vi "Test Initiate.vi"(0 "Template Tx Test in":refnum<class "niDTS BT Tx Test.lvclass">, 11 "error in (no error)":errorcluster) -> (4 "Template Tx Test out":refnum<class "niDTS BT Tx Test.lvclass">, 15 "error out":errorcluster)   [LabVIEW 2015, in "niDTS BT.lvlib" / "niDTS BT Tx Test.lvclass"]
uses:
  niDTS BT Tx Test.lvclass
  niDTS BT Tx Test.lvclass/niDTS BT Tx Test.ctl
  Instrument/INSTR TX/niDTS BT INSTR TX.lvclass
  Framework/Dut/Objects/BASE_class/niDTS Dut.lvclass
  RiviInstDriver/niRfsaBT/Objects/niRfsaBt.lvclass
  niDTS BT.lvlib
  Dut/Objects/BASE_class/niDTS BT Dut.lvclass
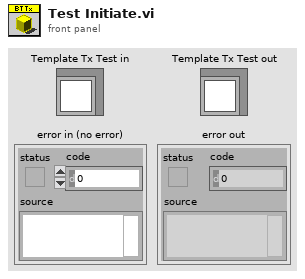
[diagram p1: front panel]
types:
  T1 = typedef "niDTS BT.lvlib/niDTS BT Tx Test INC Parameters.ctl" = cluster{"Channel":i32, "Data Rate ":i32, "Dut Tx Power":dbl, "External Attenuation (dB)":dbl[], "Auto Level":bool, "Packet type":T2, "Payload Pattern":T3, "Burst Sync":enum16{"NONE", "PREamble"}, "BD ADDRESS":u32, "Packet Length, bytes":i32, "ModAcc Measurement Paramaters":cluster{"ModAcc Enable":bool, "CFO Enable":bool, "Character Select":T4, "Averages":i32, "Averaging Mode":enum16{"RMS", "LOG", "SCALAR", "MAX", "MIN", "VECTOR"}, "Measurement Length":i32, "Measurement Offset":i32}, "OBW Measurement Parameters":T5, "TXP Measurement Parameters":T6, "IBE  Measurement Parameters":T7, "Trace Enable":bool, "Trigger":T8}
  T2 = typedef "niDTS BT.lvlib/niDTS BT INC Packet Type.ctl" = enum16{"NULL", "POLL", "FHS", "DM1", "DH1", "HV1", "HV2", "HV3", "EV3", "DV", "AUX1", "DM3", "DH3", "EV4", "EV5", "DM5", "DH5", "LE-TP"}
  T3 = typedef "niDTS BT.lvlib/niDTS BT Tx Test INC BD Payload Data.ctl" = enum16{"0", "1", "01", "00001111", "PN9", "AUTO"}
  T4 = typedef "niDTS BT.lvlib/niDTS BT Tx Test INC Modulation Characteristics.ctl" = enum16{"DF1", "DF2", "BOTH"}
  T5 = typedef "niDTS BT.lvlib/niDTS BT INC OBW Measurement Parameters.ctl" = cluster{"OBW Enable":bool, "OBW Averages":i32, "Averaging Type":enum16{"RMS", "LOG", "SCALAR", "MAX", "MIN", "VECTOR"}, "Measurement Interval Mode":enum16{"AUTO", "MANUAL"}, "Measurement Interval Length (sec)":dbl}
  T6 = typedef "niDTS BT.lvlib/niDTS BT INC TXP Measurement Parameters.ctl" = cluster{"TXP Power Enable":bool, "TXP Averages":i32, "Averaging Type":enum16{"RMS", "LOG", "SCALAR", "MAX", "MIN"}}
  T7 = typedef "niDTS BT.lvlib/niDTS BT INC EDR IBE Measurement Parameters.ctl" = cluster{"IBE Enable":bool, "IBE Averages":i32, "Averaging Type":enum16{"RMS", "LOG", "SCALAR", "MAX", "MIN", "VECTOR"}, "Numbe of Channels":i32, "Channel Mode":enum16{"InBand", "Centered"}, "Measurement Interval Mode":enum16{"AUTO", "MANUAL"}, "Measurement Interval Length (sec)":dbl}
  T8 = typedef "niDTS BT.lvlib/niDTS BT DUT INC Trigger.ctl" = cluster{"MinQuietTimeDuration (sec)":dbl, "TriggerDelay (sec)":dbl, "TriggerEdge":enum16{"RISing", "FALLing"}, "TriggerSource":enum16{"IMMediate", "RF0", "PFI0", "PFI1", "RTS0", "RTS1", "RTS2", "RTS3", "RTS4", "RTS5", "RTS6", "RTS7", "PXIStar", "SOFT"}, "TriggerThreshold (dB)":dbl, "TriggerTimeout (sec)":dbl}
  T9 = typedef "niDTS Framework.lvlib/niDTS Dut INC Handle.ctl" = refnum<data-value>
  T10 = typedef "niDTS BT.lvlib/niDTS BT Dut INC Handle.ctl" = refnum<data-value>
  T11 = typedef "niRfsaBT.lvclass/niRfsaBT INC Handle.ctl" = refnum<data-value>
  T12 = typedef "niDTS BT.lvlib/niDTS BT DUT INC Parameters.ctl" = cluster{"Channel":i32, "Pattern":enum16{"0", "1", "01", "00001111", "PN9"}, "Packet type":enum16{"NULL", "POLL", "FHS", "DM1", "DH1", "HV1", "HV2", "HV3", "EV3", "DV", "AUX1", "DM3", "DH3", "EV4", "EV5", "DM5", "DH5", "LE-TP"}, "Power":dbl, "Report Period (ms)":dbl, "BD Address":i64, "Data Rate":enum16{"1", "2", "3"}, "Number of Packets":i32, "Packet Length, bytes":i32}
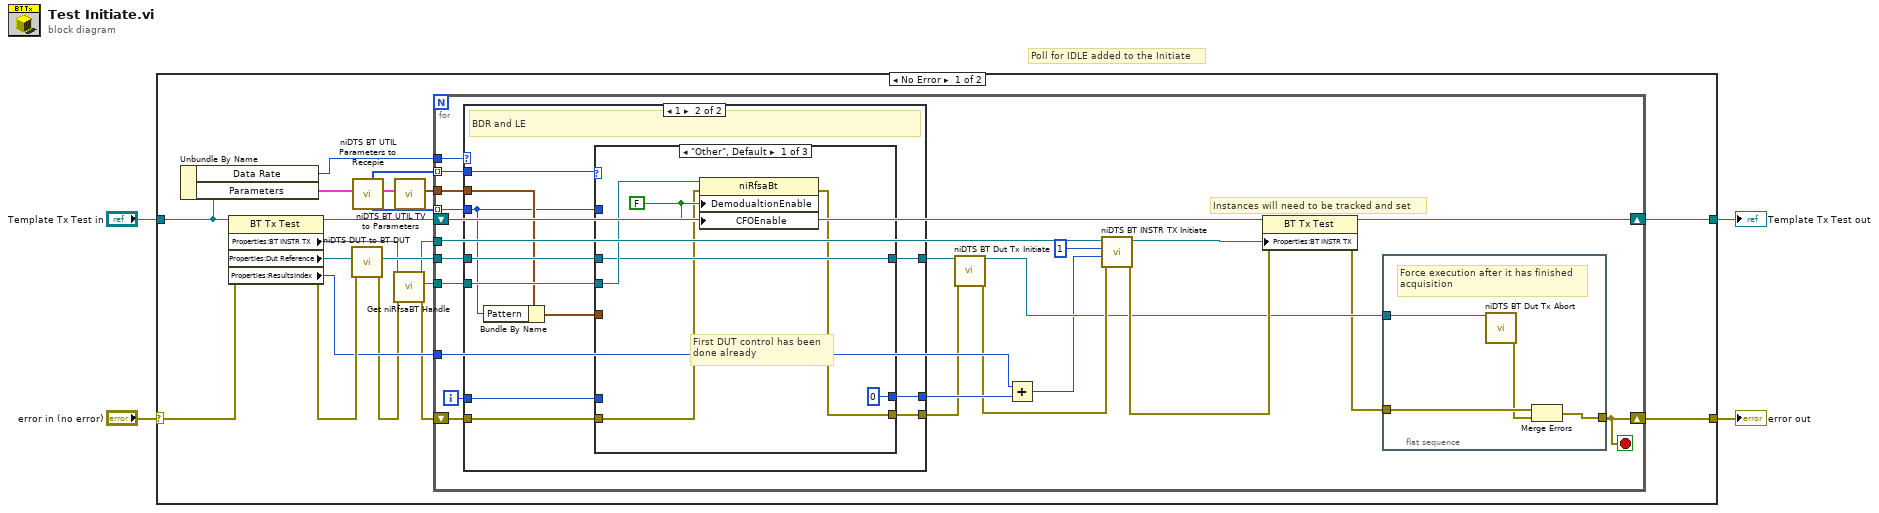
[diagram p0: block diagram]
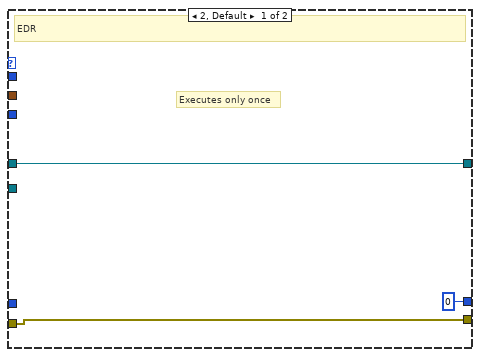
[diagram p2: hidden frame]
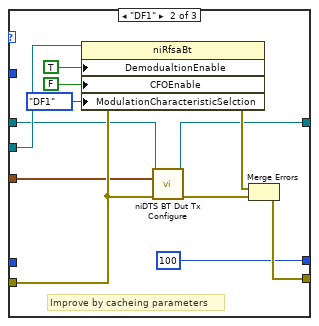
[diagram p3: hidden frame]
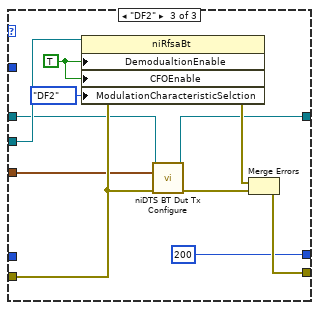
[diagram p4: hidden frame]
diagram:
  # "Poll for IDLE added to the Initiate"
  n1 = case shown="No Error" "error in (no error)" {
    selector: "error in (no error)" -> [w24 w96]
    tunnel: [w17 w96] -> w3
    tunnel: [w20 w95] -> w1
    tunnel: "Template Tx Test in" -> [w16 w95]
    frame No Error {
      n2 = Unbundle By Name(w16) -> ("Data Rate"=w5:i32, "Parameters"=w15:T1)
      n3 = property class="BT Tx Test"(reference=w16, error in=w24) -> (reference out=w21:refnum<class "niDTS BT Tx Test.lvclass">, error out=w22:errorcluster, "Properties:BT INSTR TX"=w6:refnum<class "niDTS BT INSTR TX.lvclass">, "Properties:Dut Reference"=w23:T9, "Properties:ResultsIndex"=w19:u8)
      n4 = call "niDTS DUT to BT DUT.vi"("error in"=w22, "Dut Handle"=w23) -> ("error out"=w8:errorcluster, "BT Dut Handle"=w18:T10)  [unwired: 8 in]
      n5 = call "niDTS BT UTIL Parameters to Recepie.vi"("BT Tx Parameters"=w15) -> ("BT Tx Parameters Out"=w10:T1, "Payloads"=w11:T3[], "Measurements"=w12:enum16{"Other", "DF1", "DF2"}[])  [unwired: 8 in]
      n6 = call-dynamic "Get niRfsaBT Handle.vi"("error in (no error)"=w8, "niDTS BT INSTR TX in"=w6) -> ("error out"=w7:errorcluster, "InstDriver Handle in"=w13:T11, "niDTS BT INSTR TX out"=w14:refnum<class "niDTS BT INSTR TX.lvclass">)  [unwired: 7 in]
      n7 = call "niDTS BT UTIL TV to Parameters.vi"("BT Tx Parameters"=w10) -> ("niDTS BT DUT Parameters"=w9:T12)  [unwired: 10 in]
      n8 = for {
        tunnel: w14 -> [w36]
        tunnel: w19 -> [w43]
        tunnel: w18 -> [w42]
        shift-right: [w46] -> w20
        shift-left: w21 -> [w47]
        shift-right: [w26] -> w17
        shift-left: w7 -> [w40]
        tunnel: w12 -> [w38] mode=indexing
        tunnel: w13 -> [w37]
        tunnel: w11 -> [w34] mode=indexing
        tunnel: w9 -> [w35]
        tunnel: w5 -> [w25]
        i -> [w45]
        stop <- w26 stop-if-true
        # "Instances will need to be tracked and set"
        n9 = case shown="1" w25 {
          tunnel: w45 -> [_ w61]
          tunnel: [0 w60] -> w44
          tunnel: w42 -> [w50 w59]
          tunnel: [w50 w58] -> w41
          tunnel: w40 -> [w49 w57]
          tunnel: [w49 w56] -> w39
          tunnel: w38 -> [_ w55]
          tunnel: w37 -> [_ w54]
          tunnel: w35 -> [_ w53]
          tunnel: w34 -> [_ w51]
          frame 2, Default {
            # "Executes only once"
            # "EDR"
          }
          frame 1 {
            # "BDR and LE"
            n10 = Bundle By Name(cluster=w53, "Pattern"=w51) -> (w52:T12)
            n11 = case shown="\"Other\", Default" w55 {
              tunnel: w61 -> [_ _ _]
              tunnel: [0 100 200] -> w60
              tunnel: w59 -> [w65 w72 w83]
              tunnel: [w65 w71 w82] -> w58
              tunnel: w57 -> [w64 w74 w85]
              tunnel: [w63 w75 w86] -> w56
              tunnel: w54 -> [w67 w79 w90]
              tunnel: w51 -> [_ _ _]
              tunnel: w52 -> [_ w73 w84]
              frame "Other", Default {
                w66 = FALSE ("CONFigure:RFSA:BLUetooth:MEASurement:MODulation:DemodualtionEnable")
                # "First DUT control has been\ndone already"
                n12 = property class="niRfsaBt"(reference=w67, error in=w64, "DemodualtionEnable"=w66, "CFOEnable"=w66) -> (error out=w63:errorcluster)  [unwired: 1 out]
              }
              frame "DF1" {
                # "Improve by cacheing parameters"
                n13 = property class="niRfsaBt"(reference=w79, error in=w74, "DemodualtionEnable"=TRUE ("CONFigure:RFSA:BLUetooth:MEASurement:MODulation:DemodualtionEnable"), "CFOEnable"=FALSE ("CONFigure:RFSA:BLUetooth:MEASurement:MODulation:FSK:CFO:CFOEnable"), "ModulationCharacteristicSelction"=enum16{"DF1", "DF2"}."DF1" ("CONFigure:RFSA:BLUetooth:MEASurement:MODulation:FSK:CHARacter:ModulationCharacteristicSelction")) -> (error out=w76:errorcluster)  [unwired: 1 out]
                n14 = call "niDTS BT Dut Tx Configure.vi"("Dut Handle in"=w72, "niDTS BT DUT Parameters"=w73, "error in (no error)"=w74) -> ("Dut Handle"=w71:T9, "error out"=w77:errorcluster)  [unwired: 11 in]
                n15 = Merge Errors(w76, w77) -> (w75:errorcluster)
              }
              frame "DF2" {
                w89 = TRUE ("CONFigure:RFSA:BLUetooth:MEASurement:MODulation:DemodualtionEnable")
                n16 = property class="niRfsaBt"(reference=w90, error in=w85, "DemodualtionEnable"=w89, "CFOEnable"=w89, "ModulationCharacteristicSelction"=enum16{"DF1", "DF2"}."DF2" ("CONFigure:RFSA:BLUetooth:MEASurement:MODulation:FSK:CHARacter:ModulationCharacteristicSelction")) -> (error out=w87:errorcluster)  [unwired: 1 out]
                n17 = call "niDTS BT Dut Tx Configure.vi"("Dut Handle in"=w83, "niDTS BT DUT Parameters"=w84, "error in (no error)"=w85) -> ("Dut Handle"=w82:T9, "error out"=w88:errorcluster)  [unwired: 11 in]
                n18 = Merge Errors(w87, w88) -> (w86:errorcluster)
              }
            }
          }
        }
        n19 = call "niDTS BT Dut Tx Initiate.vi"("Dut Handle in"=w41, "error in (no error)"=w39) -> ("Dut Handle out"=w29:T9, "error out"=w31:errorcluster)  [unwired: 12 in]
        n20 = Add(x=w43, y=w44) -> (x+y=w27:i32)
        n21 = call-dynamic "niDTS BT INSTR TX Initiate.vi"("error in (no error)"=w31, "Result Instance"=w27, "Driver Instance"=1, "niDTS BT INSTR TX in"=w36) -> ("error out"=w32:errorcluster, "niDTS BT INSTR TX out"=w33:refnum<class "niDTS BT INSTR TX.lvclass">)  [unwired: 6 in]
        n22 = property class="BT Tx Test"(reference=w47, error in=w32, "Properties:BT INSTR TX"=w33) -> (reference out=w46:refnum<class "niDTS BT Tx Test.lvclass">, error out=w28:errorcluster)
        n23 = flat-sequence {
          tunnel: [w94] -> w26
          tunnel: w29 -> [w93]
          tunnel: w28 -> [w92]
          frame #0 {
            # "Force execution after it has finished\nacquisition"
            n24 = call "niDTS BT Dut Tx Abort.vi"("BT Dut Handle in"=w93) -> ("error out"=w91:errorcluster)  [unwired: 13 in, 1 out]
            n25 = Merge Errors(w92, w91) -> (w94:errorcluster)
          }
        }
      }
    }
    frame Error {
    }
  }
  "error out" <- w3
  "Template Tx Test out" <- w1
